vi "Read Type.vi"(8 "Error In":errorcluster, 11 "InvertedSection In":refnum<class "InvertedSection.lvclass">) -> (0 "Error Out":errorcluster, 2 "Type":T1=enum."Unknown", 3 "InvertedSection Out":refnum<class "InvertedSection.lvclass">)   [LabVIEW 2018, in "Toolkit.lvlib" / "Tokens.lvlib" / "InvertedSection.lvclass"]
doc: "Gets the Token type. LabVIEW 2009 does not have the Get LV Class Name function, so this is a workaround to determine the Node class/type during run-time."
uses:
  InvertedSection.lvclass
  Type Definitions/Types.ctl
  Tokens.lvlib
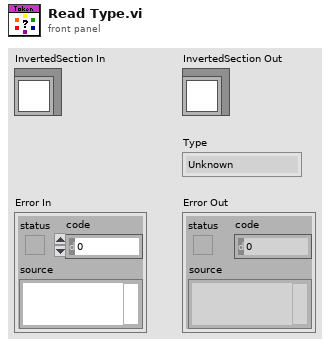
[diagram p1: front panel]
types:
  T1 = typedef "Toolkit.lvlib/Tokens.lvlib/Types.ctl" = enum16{"Begin Section", "Comment", "End Section", "Escaped Variable", "Inverted Section", "Partial", "Set Delimiter", "Text", "Unescaped Variable", "Unknown"}
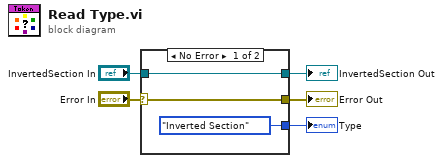
[diagram p0: block diagram]
diagram:
  n1 = case shown="No Error" "Error In" {
    selector: "Error In" -> [w8 w9]
    tunnel: [w8 w9] -> w2
    tunnel: "InvertedSection In" -> [w7 w10]
    tunnel: [w7 w10] -> w1
    tunnel: [Types."Inverted Section" ("Type") _] -> w3
    frame No Error {
    }
    frame Error {
    }
  }
  "Error Out" <- w2
  "InvertedSection Out" <- w1
  "Type" <- w3
